vi "CalcCameraFlex.vi"(2 "Camera Target":dbl, 3 "B1":dbl, 4 "Rotator Position":dbl) -> (0 "Camera Flex Target":dbl, 1 "Flex":dbl)   [LabVIEW 2015]
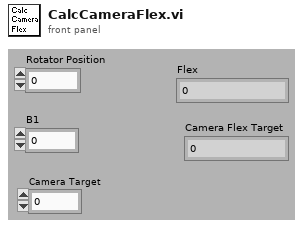
[diagram p1: front panel]
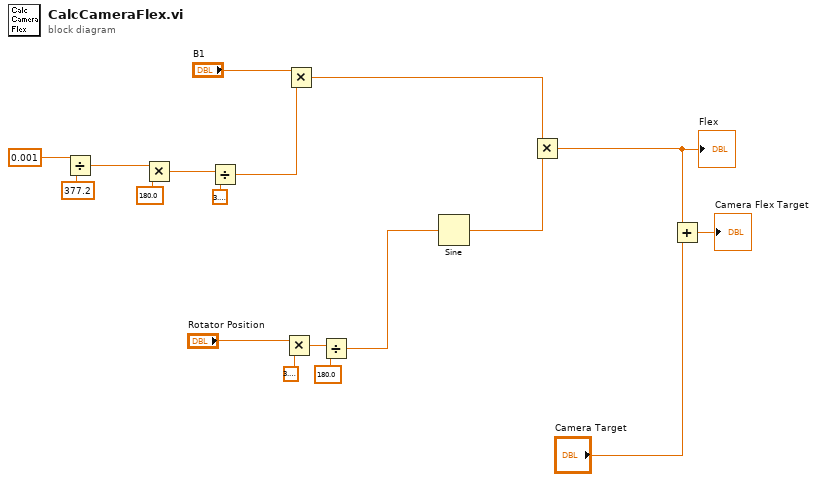
[diagram p0: block diagram]
diagram:
  n1 = Divide(x=0.001, y=377.2) -> (x/y=w10:dbl)
  n2 = Multiply(x=w10, y=180.0) -> (x*y=w8:dbl)
  n3 = Divide(x=w8, y=3.141592653589793) -> (x/y=w6:dbl)
  n4 = Multiply(x="Rotator Position", y=3.141592653589793) -> (x*y=w16:dbl)
  n5 = Multiply(x="B1", y=w6) -> (x*y=w5:dbl)
  n6 = Divide(x=w16, y=180.0) -> (x/y=w14:dbl)
  n7 = Sine(x=w14) -> (sin(x)=w4:dbl)
  n8 = Multiply(x=w5, y=w4) -> (x*y=w3:dbl)
  "Flex" <- w3
  n9 = Add(x=w3, y="Camera Target") -> (x+y=→"Camera Flex Target":dbl)
